vi "SW_Load_settings_to_main_tab_3.vi"(0 "Settings path in":path, 2 "Researcher name":string="Researcher", 3 "error in (no error)":errorcluster) -> (6 "Settings cluster out":T1={"Defaults"={"Default User"=0.0, "VISA Resource Name "="", "Histogram parameters"={"max"=300.0, "min"=0.0, "# bins"=10, "threshold"=8.0, "thr. type"=enum."higher accepted"}}, "Recording and saving"={"Researcher name"="", "Name prefix"="", "Data post-processing"={"Filter type"=enum."Savitzky-Golay", "Length"=31, "Order"=3}, "Stop at"=0.0, "\"Stop at\" enabled"=FALSE, "Default save folder path"=path "", "Acquisition FPS"=enum."Max"}, "Geometry"={"Cage diameter, mm"=0, "Starting angle MIDFIELD"=0, "Starting angle BORDER"=0, "Radius, mm CENTER"=0, "Radius, mm MIDFIELD"=0, "N segments MIDFIELD"=0, "N segments BORDER"=0, "R-gap, mm"=0.0, "Bridge swap"=FALSE, "Bridge H. offset"=0.0, "Bridge V. offset"=0.0, "Twisted neck"=FALSE, "Alt. magn. orientation"=FALSE, "Sensor board size"=enum."Small"}, "IO parameters"={"IO general config."=0, "IO 1 configuration"=0, "IO 2 configuration"=0, "IO 3 configuration"=0, "IO 4 configuration"=0, "Activate ext. RS-232"=0, "IO inversion config."=0, "Sync capability"=1}, "Conditions presets array"=[{"Enabled"=FALSE, "Name"="", "Specifier(s)"=[], "Response"={"Response type"=enum."Air puff", "TTL port"=enum."Port 1", "TTL pulse length, ms"=0.0}, "Has been set"=FALSE}, {"Enabled"=FALSE, "Name"="", "Specifier(s)"=[], "Response"={"Response type"=enum."Air puff", "TTL port"=enum."Port 1", "TTL pulse length, ms"=0.0}, "Has been set"=FALSE}, {"Enabled"=FALSE, "Name"="", "Specifier(s)"=[], "Response"={"Response type"=enum."Air puff", "TTL port"=enum."Port 1", "TTL pulse length, ms"=0.0}, "Has been set"=FALSE}, {"Enabled"=FALSE, "Name"="", "Specifier(s)"=[], "Response"={"Response type"=enum."Air puff", "TTL port"=enum."Port 1", "TTL pulse length, ms"=0.0}, "Has been set"=FALSE}, {"Enabled"=FALSE, "Name"="", "Specifier(s)"=[], "Response"={"Response type"=enum."Air puff", "TTL port"=enum."Port 1", "TTL pulse length, ms"=0.0}, "Has been set"=FALSE}, {"Enabled"=FALSE, "Name"="", "Specifier(s)"=[], "Response"={"Response type"=enum."Air puff", "TTL port"=enum."Port 1", "TTL pulse length, ms"=0.0}, "Has been set"=FALSE}, {"Enabled"=FALSE, "Name"="", "Specifier(s)"=[], "Response"={"Response type"=enum."Air puff", "TTL port"=enum."Port 1", "TTL pulse length, ms"=0.0}, "Has been set"=FALSE}, {"Enabled"=FALSE, "Name"="", "Specifier(s)"=[], "Response"={"Response type"=enum."Air puff", "TTL port"=enum."Port 1", "TTL pulse length, ms"=0.0}, "Has been set"=FALSE}, {"Enabled"=FALSE, "Name"="", "Specifier(s)"=[], "Response"={"Response type"=enum."Air puff", "TTL port"=enum."Port 1", "TTL pulse length, ms"=0.0}, "Has been set"=FALSE}, {"Enabled"=FALSE, "Name"="", "Specifier(s)"=[], "Response"={"Response type"=enum."Air puff", "TTL port"=enum."Port 1", "TTL pulse length, ms"=0.0}, "Has been set"=FALSE}, {"Enabled"=FALSE, "Name"="", "Specifier(s)"=[], "Response"={"Response type"=enum."Air puff", "TTL port"=enum."Port 1", "TTL pulse length, ms"=0.0}, "Has been set"=FALSE}, {"Enabled"=FALSE, "Name"="", "Specifier(s)"=[], "Response"={"Response type"=enum."Air puff", "TTL port"=enum."Port 1", "TTL pulse length, ms"=0.0}, "Has been set"=FALSE}, {"Enabled"=FALSE, "Name"="", "Specifier(s)"=[], "Response"={"Response type"=enum."Air puff", "TTL port"=enum."Port 1", "TTL pulse length, ms"=0.0}, "Has been set"=FALSE}, {"Enabled"=FALSE, "Name"="", "Specifier(s)"=[], "Response"={"Response type"=enum."Air puff", "TTL port"=enum."Port 1", "TTL pulse length, ms"=0.0}, "Has been set"=FALSE}], "Calibration parameters"={"Timing calibration sw/hw"=1.0, "True FPS"=80.0, "True frame time, s"=80.0, "Disp. calibration info"=[]}, "Settings loaded OK"=FALSE} {"Calibration parameters"."True frame time, s" format="%.10g"; "Calibration parameters"."Disp. calibration info"."Speed, µl per ms" format="%.3g"; "Calibration parameters"."True FPS" format="%.10g"; "Calibration parameters"."Timing calibration sw/hw" format="%.10g"; "Conditions presets array"."Specifier(s)"."Validity criteria(s)"."Validity value" min=0.0 step=0.1 format="%.2g"; "Conditions presets array"."Specifier(s)"."Value" step=1.0 format="%#.2g"; "Recording and saving"."Data post-processing"."Order" min=3 max=11 step=2; "Recording and saving"."Data post-processing"."Length" min=5 max=301 step=2; "Geometry"."Cage diameter, mm" scale=0.0..340.0}, 7 "Settings file path out":path, 10 "error out":errorcluster={"status"=TRUE, "code"=1, "source"="Dequeue Element in NI_LVConfig.lvlib:Read Value Without Comment.vi->NI_LVConfig.lvlib:Read Key (I32).vi->SW_Load_settings_to_main_tab.vi"})   [LabVIEW 2018, in "Tracker.lvlib"]
uses:
  Tracker.lvlib
  Controls/CTL_Settings_cluster.ctl
  Controls/CTL_Histogram_parameters.ctl
  Controls/CTL_Filter_selector.ctl
  Controls/CTL_Acquisition_speed_selector.ctl
  Controls/CTL_Segmented_plot_parameters.ctl
  Controls/CTL_IO_params_cluster.ctl
  Controls/CTL_Conditions_Array.ctl
  Controls/CTL_Conditions_Cluster.ctl
  Controls/CTL_Condition_type.ctl
  Controls/CTL_Comparison_type.ctl
  Controls/CTL_Validity_check_criteria.ctl
  Controls/CTL_Response_info.ctl
  Controls/CTL_Condition_response_type.ctl
  Controls/CTL_Reponse_port_info.ctl
  Controls/CTL_Calibration_parameters.ctl
  Controls/CTL_Dispenser_calibration_info.ctl
  Controls/CTL_Conditions_All_Presets_Cluster.ctl
  <vilib>/Utility/sysdir.llb/System Directory Type.ctl
  <vilib>/Utility/config.llb/NI_LVConfig.lvlib
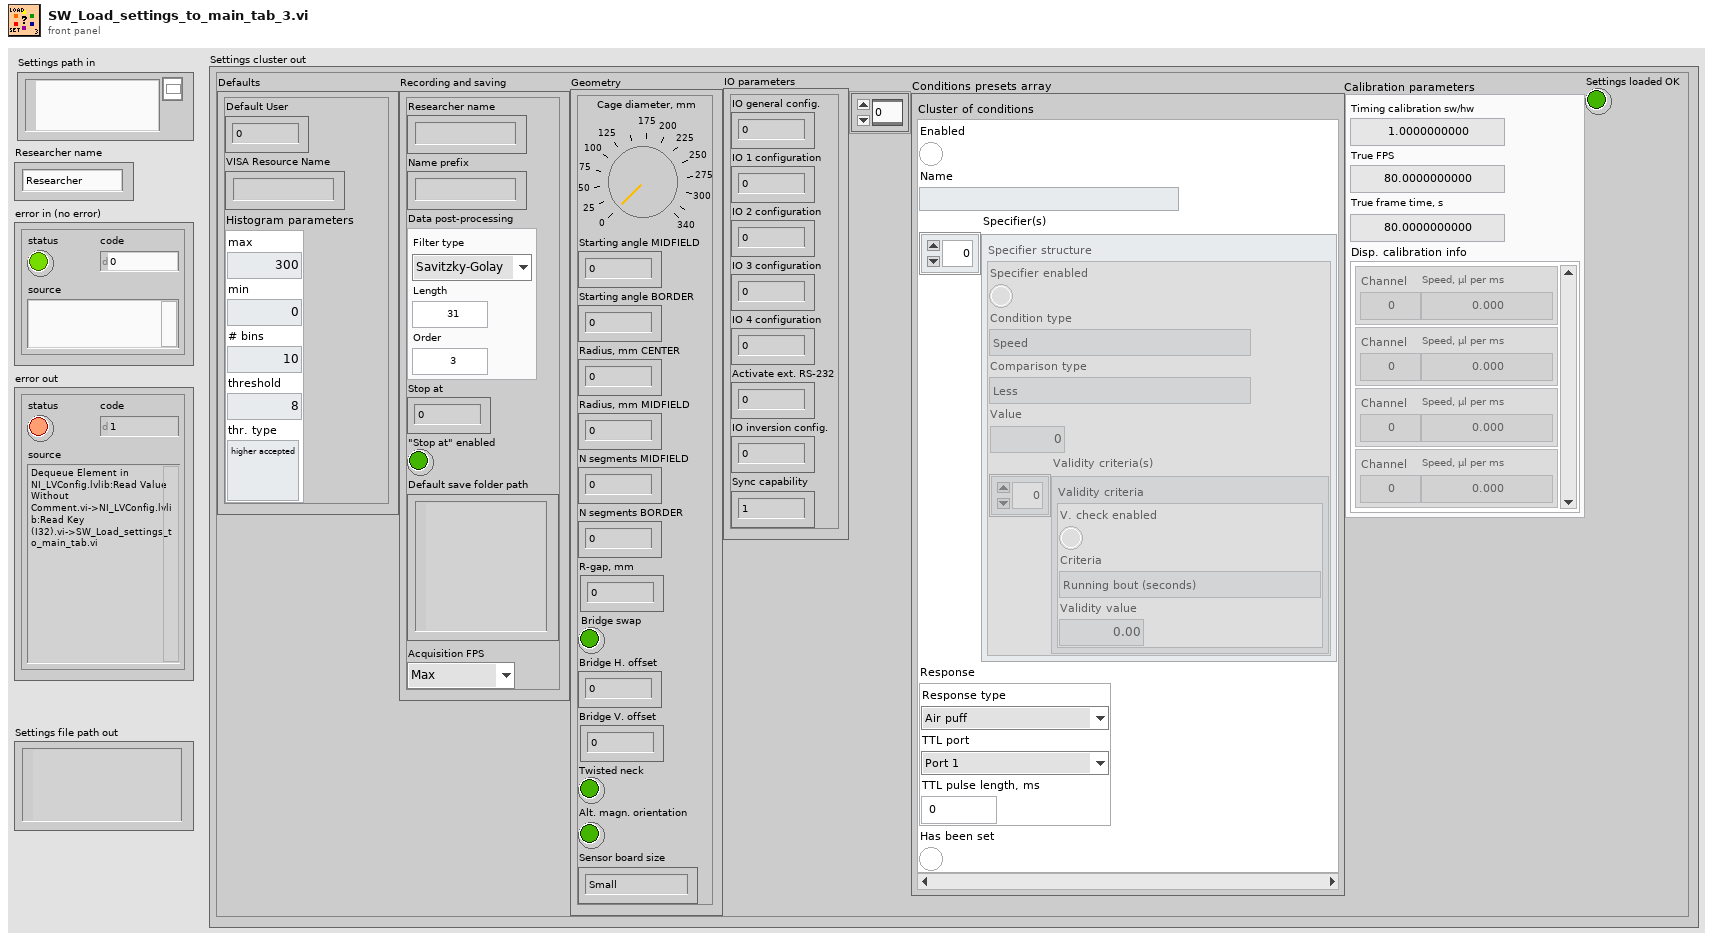
[diagram p1: front panel]
types:
  T1 = typedef "Tracker.lvlib/CTL_Settings_cluster.ctl" = cluster{"Defaults":cluster{"Default User":dbl, "VISA Resource Name ":string, "Histogram parameters":T2}, "Recording and saving":cluster{"Researcher name":string, "Name prefix":string, "Data post-processing":T3, "Stop at":dbl, "\"Stop at\" enabled":bool, "Default save folder path":path, "Acquisition FPS":T4}, "Geometry":T5, "IO parameters":T6, "Conditions presets array":T7, "Calibration parameters":T15, "Settings loaded OK":bool}
  T2 = typedef "Tracker.lvlib/CTL_Histogram_parameters.ctl" = cluster{"max":dbl, "min":dbl, "# bins":i32, "threshold":dbl, "thr. type":enum16{"higher accepted", "lower accepted"}}
  T3 = typedef "Tracker.lvlib/CTL_Filter_selector.ctl" = cluster{"Filter type":enum16{"None", "Savitzky-Golay"}, "Length":i32, "Order":i32}
  T4 = typedef "Tracker.lvlib/CTL_Acquisition_speed_selector.ctl" = enum16{"Max", "Optimal", "Eco"}
  T5 = typedef "Tracker.lvlib/CTL_Segmented_plot_parameters.ctl" = cluster{"Cage diameter, mm":u16, "Starting angle MIDFIELD":i16, "Starting angle BORDER":i16, "Radius, mm CENTER":u16, "Radius, mm MIDFIELD":u16, "N segments MIDFIELD":u8, "N segments BORDER":u8, "R-gap, mm":sgl, "Bridge swap":bool, "Bridge H. offset":sgl, "Bridge V. offset":sgl, "Twisted neck":bool, "Alt. magn. orientation":bool, "Sensor board size":enum16{"Small", "Large"}}
  T6 = typedef "Tracker.lvlib/CTL_IO_params_cluster.ctl" = cluster{"IO general config.":u16, "IO 1 configuration":u16, "IO 2 configuration":u16, "IO 3 configuration":u16, "IO 4 configuration":u16, "Activate ext. RS-232":u16, "IO inversion config.":u16, "Sync capability":u8}
  T7 = typedef "Tracker.lvlib/CTL_Conditions_Array.ctl" = T8[]
  T8 = typedef "Tracker.lvlib/CTL_Conditions_Cluster.ctl" = cluster{"Enabled":bool, "Name":string, "Specifier(s)":cluster{"Specifier enabled":bool, "Condition type":T9, "Comparison type":T10, "Value":dbl, "Validity criteria(s)":cluster{"V. check enabled":bool, "Criteria":T11, "Validity value":dbl}[]}[], "Response":T12, "Has been set":bool}
  T9 = typedef "Tracker.lvlib/CTL_Condition_type.ctl" = enum16{"Speed", "Zone", "Angle to wall"}
  T10 = typedef "Tracker.lvlib/CTL_Comparison_type.ctl" = enum16{"Less", "Less or Equal", "Equal", "Greater or Equal", "Greater", "Not Equal"}
  T11 = typedef "Tracker.lvlib/CTL_Validity_check_criteria.ctl" = enum16{"Running bout (seconds)", "Running bout (meters)"}
  T12 = typedef "Tracker.lvlib/CTL_Response_info.ctl" = cluster{"Response type":T13, "TTL port":T14, "TTL pulse length, ms":dbl}
  T13 = typedef "Tracker.lvlib/CTL_Condition_response_type.ctl" = enum16{"None", "Air puff", "Liquid reward"}
  T14 = typedef "Tracker.lvlib/CTL_Reponse_port_info.ctl" = enum16{"Port 1", "Port 2", "Port 3", "Port 4"}
  T15 = typedef "Tracker.lvlib/CTL_Calibration_parameters.ctl" = cluster{"Timing calibration sw/hw":dbl, "True FPS":dbl, "True frame time, s":dbl, "Disp. calibration info":T16}
  T16 = typedef "Tracker.lvlib/CTL_Dispenser_calibration_info.ctl" = cluster{"Channel":u8, "Speed, µl per ms":dbl}[]
  T17 = typedef "Tracker.lvlib/CTL_Conditions_All_Presets_Cluster.ctl" = cluster{"[0]":string, "[1]":string, "[2]":string, "[3]":string, "[4]":string, "[5]":string, "[6]":string, "[7]":string, "[8]":string}
  T18 = typedef "NI_LVConfig.lvlib/Config Data RefNum.ctl" = refnum<k1>
  T19 = cluster{"Default User":dbl, "VISA Resource Name ":string, "Histogram parameters":T2}
  T20 = cluster{"Researcher name":string, "Name prefix":string, "Data post-processing":T3, "Stop at":dbl, "\"Stop at\" enabled":bool, "Default save folder path":path, "Acquisition FPS":T4}
  T21 = typedef "System Directory Type.ctl" = i32
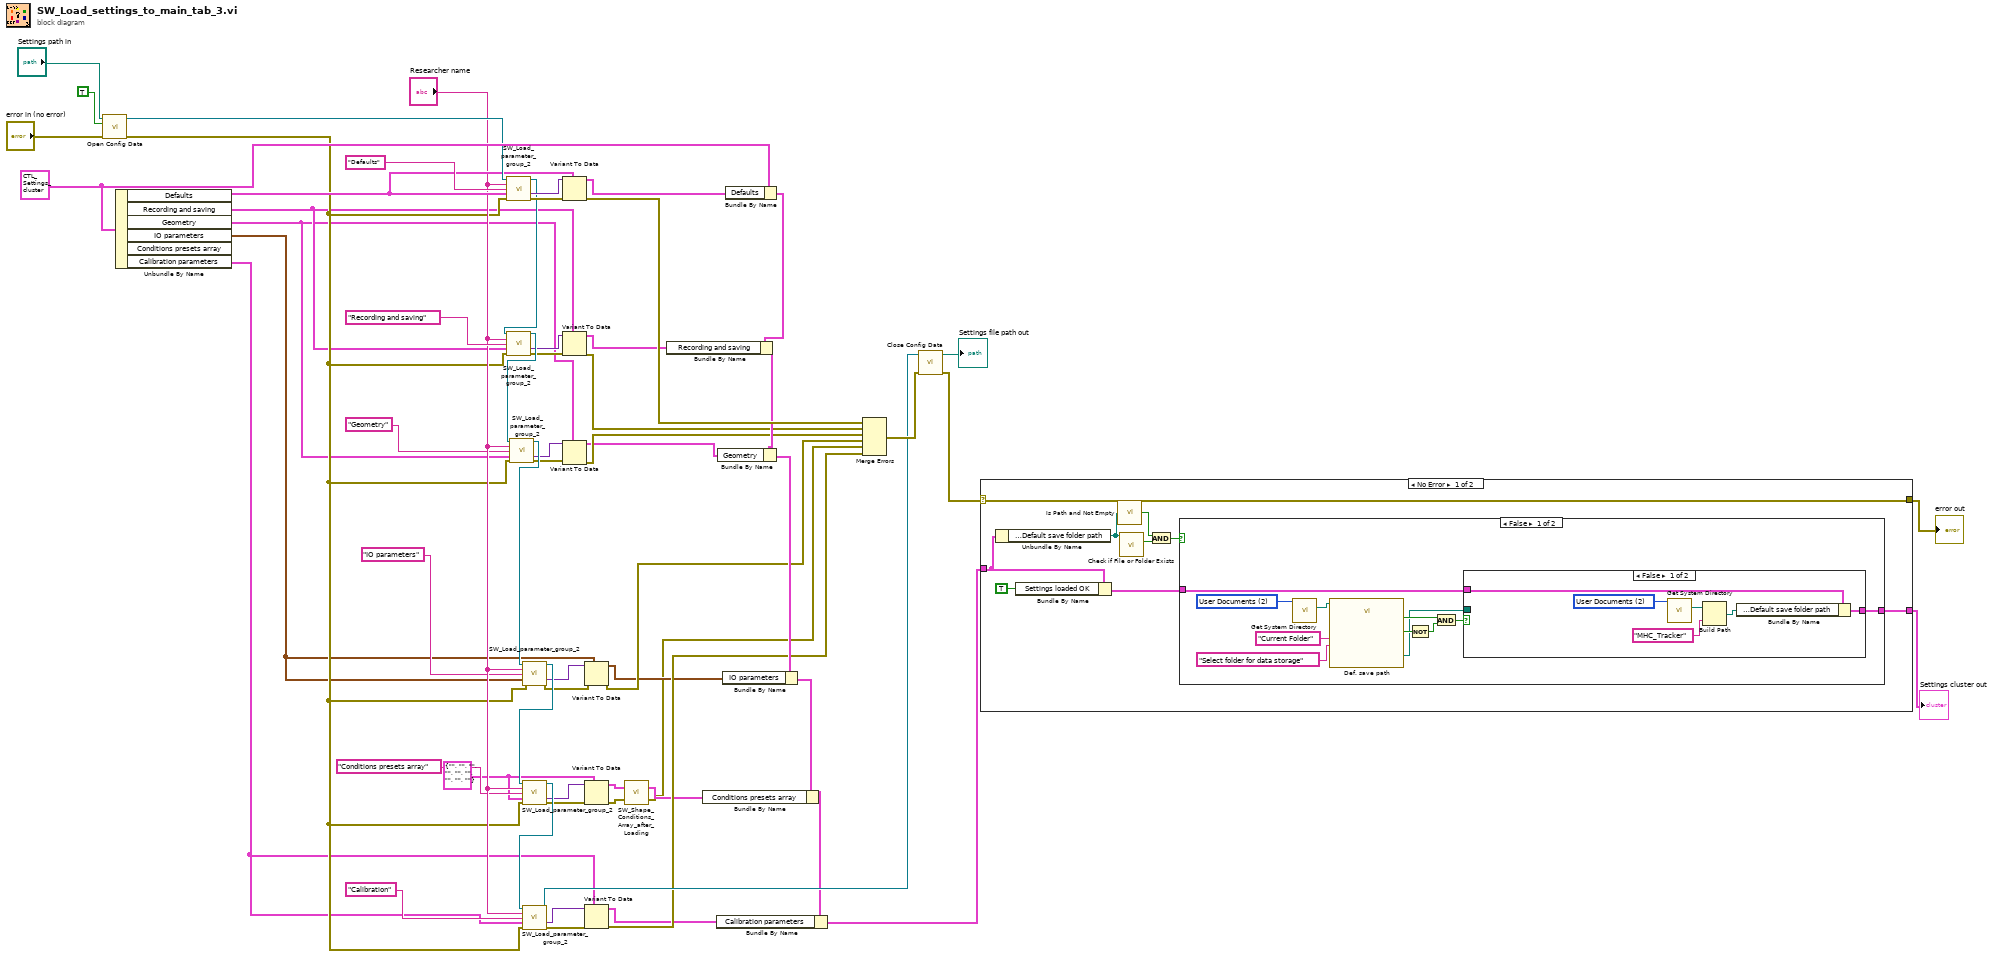
[diagram p0: block diagram]
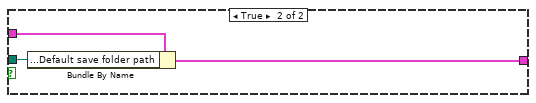
[diagram p2: hidden frame]
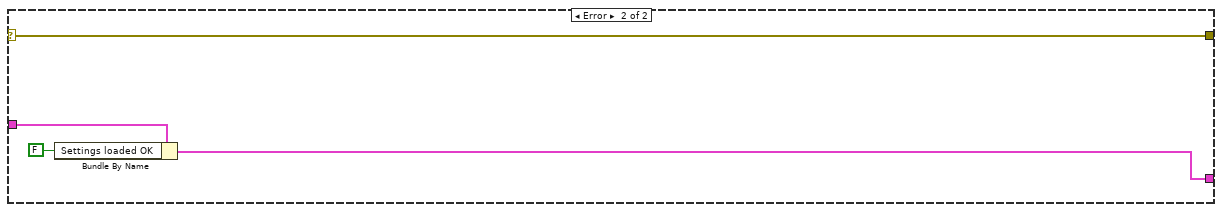
[diagram p4: hidden frame]
diagram:
  w1 = T17 {"[0]"="", "[1]"="", "[2]"="", "[3]"="", "[4]"="", "[5]"="", "[6]"="", "[7]"="", "[8]"=""} ("Condition presets prepared for saving out")
  w59 = T1 {"Defaults"={"Default User"=0.0, "VISA Resource Name "="", "Histogram parameters"={"max"=300.0, "min"=0.0, "# bins"=10, "threshold"=8.0, "thr. type"=enum."higher accepted"}}, "Recording and saving"={"Researcher name"="Researcher", "Name prefix"="Track", "Data post-processing"={"Filter type"=enum."Savitzky-Golay", "Length"=31, "Order"=3}, "Stop at"=0.0, "\"Stop at\" enabled"=FALSE, "Default save folder path"=path "", "Acquisition FPS"=enum."Max"}, "Geometry"={"Cage diameter, mm"=180, "Starting angle MIDFIELD"=0, "Starting angle BORDER"=0, "Radius, mm CENTER"=30, "Radius, mm MIDFIELD"=75, "N segments MIDFIELD"=2, "N segments BORDER"=4, "R-gap, mm"=0.0, "Bridge swap"=FALSE, "Bridge H. offset"=0.0, "Bridge V. offset"=0.0, "Twisted neck"=FALSE, "Alt. magn. orientation"=FALSE, "Sensor board size"=enum."Small"}, "IO parameters"={"IO general config."=12, "IO 1 configuration"=1, "IO 2 configuration"=1, "IO 3 configuration"=0, "IO 4 configuration"=0, "Activate ext. RS-232"=0, "IO inversion config."=0, "Sync capability"=1}, "Conditions presets array"=[{"Enabled"=FALSE, "Name"="", "Specifier(s)"=[], "Response"={"Response type"=enum."Air puff", "TTL port"=enum."Port 1", "TTL pulse length, ms"=0.0}, "Has been set"=FALSE}, {"Enabled"=FALSE, "Name"="", "Specifier(s)"=[], "Response"={"Response type"=enum."Air puff", "TTL port"=enum."Port 1", "TTL pulse length, ms"=0.0}, "Has been set"=FALSE}, {"Enabled"=FALSE, "Name"="", "Specifier(s)"=[], "Response"={"Response type"=enum."Air puff", "TTL port"=enum."Port 1", "TTL pulse length, ms"=0.0}, "Has been set"=FALSE}, {"Enabled"=FALSE, "Name"="", "Specifier(s)"=[], "Response"={"Response type"=enum."Air puff", "TTL port"=enum."Port 1", "TTL pulse length, ms"=0.0}, "Has been set"=FALSE}, {"Enabled"=FALSE, "Name"="", "Specifier(s)"=[], "Response"={"Response type"=enum."Air puff", "TTL port"=enum."Port 1", "TTL pulse length, ms"=0.0}, "Has been set"=FALSE}, {"Enabled"=FALSE, "Name"="", "Specifier(s)"=[], "Response"={"Response type"=enum."Air puff", "TTL port"=enum."Port 1", "TTL pulse length, ms"=0.0}, "Has been set"=FALSE}, {"Enabled"=FALSE, "Name"="", "Specifier(s)"=[], "Response"={"Response type"=enum."Air puff", "TTL port"=enum."Port 1", "TTL pulse length, ms"=0.0}, "Has been set"=FALSE}, {"Enabled"=FALSE, "Name"="", "Specifier(s)"=[], "Response"={"Response type"=enum."Air puff", "TTL port"=enum."Port 1", "TTL pulse length, ms"=0.0}, "Has been set"=FALSE}, {"Enabled"=FALSE, "Name"="", "Specifier(s)"=[], "Response"={"Response type"=enum."Air puff", "TTL port"=enum."Port 1", "TTL pulse length, ms"=0.0}, "Has been set"=FALSE}, {"Enabled"=FALSE, "Name"="", "Specifier(s)"=[], "Response"={"Response type"=enum."Air puff", "TTL port"=enum."Port 1", "TTL pulse length, ms"=0.0}, "Has been set"=FALSE}, {"Enabled"=FALSE, "Name"="", "Specifier(s)"=[], "Response"={"Response type"=enum."Air puff", "TTL port"=enum."Port 1", "TTL pulse length, ms"=0.0}, "Has been set"=FALSE}, {"Enabled"=FALSE, "Name"="", "Specifier(s)"=[], "Response"={"Response type"=enum."Air puff", "TTL port"=enum."Port 1", "TTL pulse length, ms"=0.0}, "Has been set"=FALSE}, {"Enabled"=FALSE, "Name"="", "Specifier(s)"=[], "Response"={"Response type"=enum."Air puff", "TTL port"=enum."Port 1", "TTL pulse length, ms"=0.0}, "Has been set"=FALSE}, {"Enabled"=FALSE, "Name"="", "Specifier(s)"=[], "Response"={"Response type"=enum."Air puff", "TTL port"=enum."Port 1", "TTL pulse length, ms"=0.0}, "Has been set"=FALSE}], "Calibration parameters"={"Timing calibration sw/hw"=1.0, "True FPS"=80.0, "True frame time, s"=80.0, "Disp. calibration info"=[{"Channel"=1, "Speed, µl per ms"=1.0}, {"Channel"=2, "Speed, µl per ms"=1.0}, {"Channel"=3, "Speed, µl per ms"=1.0}, {"Channel"=4, "Speed, µl per ms"=1.0}]}, "Settings loaded OK"=FALSE} ("Settings cluster")
  n1 = call <vilib>:"Open Config Data.vi"("error in (no error)"="error in (no error)", "create file if necessary (T)"=TRUE, "configuration file path"="Settings path in") -> ("error out"=w26:errorcluster, "refnum"=w47:T18)  [unwired: 6 in, 1 out]
  n2 = Unbundle By Name(w59) -> ("Defaults"=w43:T19, "Recording and saving"=w13:T20, "Geometry"=w11:T5, "IO parameters"=w9:T6, "Calibration parameters"=w7:T15)  [unwired: 1 out]
  n3 = call "SW_Load_parameter_group_2.vi"("Settings file refnum in"=w47, "Researcher name"="Researcher name", "Parameter group (section)"="Defaults" ("Group"), "Default value data in"=w43, "error in"=w26) -> ("Settings file refnum out"=w34:T18, "Group (section) cluster data out"=w44:variant, "error out"=w46:errorcluster)  [unwired: 8 in]
  n4 = call "SW_Load_parameter_group_2.vi"("Settings file refnum in"=w34, "Researcher name"="Researcher name", "Parameter group (section)"="Recording and saving" ("Group"), "Default value data in"=w13, "error in"=w26) -> ("Settings file refnum out"=w33:T18, "Group (section) cluster data out"=w25:variant, "error out"=w27:errorcluster)  [unwired: 8 in]
  n5 = call "SW_Load_parameter_group_2.vi"("Settings file refnum in"=w33, "Researcher name"="Researcher name", "Parameter group (section)"="Geometry" ("Group"), "Default value data in"=w11, "error in"=w26) -> ("Settings file refnum out"=w32:T18, "Group (section) cluster data out"=w23:variant, "error out"=w24:errorcluster)  [unwired: 8 in]
  n6 = call "SW_Load_parameter_group_2.vi"("Settings file refnum in"=w32, "Researcher name"="Researcher name", "Parameter group (section)"="IO parameters" ("Group"), "Default value data in"=w9, "error in"=w26) -> ("Settings file refnum out"=w31:T18, "Group (section) cluster data out"=w16:variant, "error out"=w28:errorcluster)  [unwired: 8 in]
  n7 = call "SW_Load_parameter_group_2.vi"("Settings file refnum in"=w31, "Researcher name"="Researcher name", "Parameter group (section)"="Conditions presets array" ("Group"), "Default value data in"=w1, "error in"=w26) -> ("Settings file refnum out"=w30:T18, "Group (section) cluster data out"=w15:variant, "error out"=w21:errorcluster)  [unwired: 8 in]
  n8 = call "SW_Load_parameter_group_2.vi"("Settings file refnum in"=w30, "Researcher name"="Researcher name", "Parameter group (section)"="Calibration" ("Group"), "Default value data in"=w7, "error in"=w26) -> ("Settings file refnum out"=w51:T18, "Group (section) cluster data out"=w14:variant, "error out"=w22:errorcluster)  [unwired: 8 in]
  n9 = Variant To Data(error in=w46, type=w43, Variant=w44) -> (data=w42:T19, error out=w45:errorcluster)
  n10 = Variant To Data(error in=w27, type=w13, Variant=w25) -> (data=w12:T20, error out=w20:errorcluster)
  n11 = Variant To Data(error in=w24, type=w11, Variant=w23) -> (data=w10:T5, error out=w19:errorcluster)
  n12 = Variant To Data(error in=w28, type=w9, Variant=w16) -> (data=w8:T6, error out=w18:errorcluster)
  n13 = Variant To Data(error in=w21, type=w1, Variant=w15) -> (data=w4:T17, error out=w5:errorcluster)
  n14 = Variant To Data(error in=w22, type=w7, Variant=w14) -> (data=w6:T15, error out=w17:errorcluster)
  n15 = call "SW_Shape_Conditions_Array_after_Loading.vi"("error in (no error)"=w5, "Condition presets loaded in"=w4) -> ("error out"=w2:errorcluster, "Conditions presets array out"=w3:T7)
  n16 = Bundle By Name(cluster=w59, "Defaults"=w42) -> (w41:T1)
  n17 = Bundle By Name(cluster=w41, "Recording and saving"=w12) -> (w29:T1)
  n18 = Bundle By Name(cluster=w29, "Geometry"=w10) -> (w58:T1)
  n19 = Bundle By Name(cluster=w58, "IO parameters"=w8) -> (w57:T1)
  n20 = Bundle By Name(cluster=w57, "Conditions presets array"=w3) -> (w50:T1)
  n21 = Bundle By Name(cluster=w50, "Calibration parameters"=w6) -> (w49:T1)
  n22 = Merge Errors(w45, w20, w19, w18, w2, w17) -> (w56:errorcluster)
  n23 = call <vilib>:"Close Config Data.vi"("error in (no error)"=w56, "refnum"=w51) -> ("error out"=w55:errorcluster, "file path"=→"Settings file path out":path)  [unwired: 8 in]
  n24 = case shown="No Error" w55 {
    selector: w55 -> [w70 w94]
    tunnel: [w70 w94] -> w54
    tunnel: w49 -> [w69 w96]
    tunnel: [w63 w93] -> w53
    frame No Error {
      n25 = Unbundle By Name(w69) -> ("Recording and saving.Default save folder path"=w67:path)
      n26 = Bundle By Name(cluster=w69, "Settings loaded OK"=TRUE) -> (w64:T1)
      n27 = call <vilib>:"Is Path and Not Empty.vi"("path"=w67) -> ("Is Path and Not Empty?"=w68:bool)  [unwired: 4 in]
      n28 = call <vilib>:"Check if File or Folder Exists.vi"("path"=w67) -> ("file or folder exists?"=w66:bool)  [unwired: 8 in, 2 out]
      n29 = And(x=w68, y=w66) -> (x .and. y?=w65:bool)
      n30 = case shown="False" w65 {
        tunnel: w64 -> [w74 w92]
        tunnel: [w73 w92] -> w63
        frame False {
          w81 = T21 2 items=["User Home"=0, "User Desktop"=1, "User Documents"=2, "User Application Data"=3, "User Preferences"=4, "User Temporary"=5, "Public Documents"=6, "Public Application Data"=7, "Public Preferences"=8, "Public Cache"=13, "System Core Libraries"=9, "System Installed Libraries"=10, "Application Files"=11, "Boot Volume Root"=12] ("system directory type")
          n31 = call <vilib>:"Get System Directory.vi"("system directory type"=w81) -> ("system directory"=w82:path)  [unwired: 10 in]
          n32 = call "Def. save path"("start path"=w82, "prompt"="Select folder for data storage", "button label"="Current Folder") -> ("selected path"=w72:path, "exists"=w76:bool, "cancelled"=w78:bool)  [unwired: 9 in, 1 out]
          n33 = Not(x=w78) -> (.not. x?=w77:bool)
          n34 = And(x=w76, y=w77) -> (x .and. y?=w75:bool)
          n35 = case shown="False" w75 {
            tunnel: w74 -> [w84 w91]
            tunnel: [w83 w90] -> w73
            tunnel: w72 -> [_ w89]
            frame False {
              w87 = T21 2 items=["User Home"=0, "User Desktop"=1, "User Documents"=2, "User Application Data"=3, "User Preferences"=4, "User Temporary"=5, "Public Documents"=6, "Public Application Data"=7, "Public Preferences"=8, "Public Cache"=13, "System Core Libraries"=9, "System Installed Libraries"=10, "Application Files"=11, "Boot Volume Root"=12] ("system directory type")
              n36 = call <vilib>:"Get System Directory.vi"("system directory type"=w87) -> ("system directory"=w88:path)  [unwired: 10 in]
              n37 = Build Path(base path=w88, name or relative path="MHC_Tracker") -> (appended path=w86:path)
              n38 = Bundle By Name(cluster=w84, "Recording and saving.Default save folder path"=w86) -> (w83:T1)
            }
            frame True {
              n39 = Bundle By Name(cluster=w91, "Recording and saving.Default save folder path"=w89) -> (w90:T1)
            }
          }
        }
        frame True {
        }
      }
    }
    frame Error {
      n40 = Bundle By Name(cluster=w96, "Settings loaded OK"=FALSE) -> (w93:T1)
    }
  }
  "Settings cluster out" <- w53
  "error out" <- w54
